vi "Prograss Bar Caller.vi"(8 "error in":errorcluster, 10 "Progress bar window values input":T1) -> (0 "error out":errorcluster)   [LabVIEW 2020]
uses:
  Progress bar window values input cluster.ctl
  Global Variables/General Globals.vi
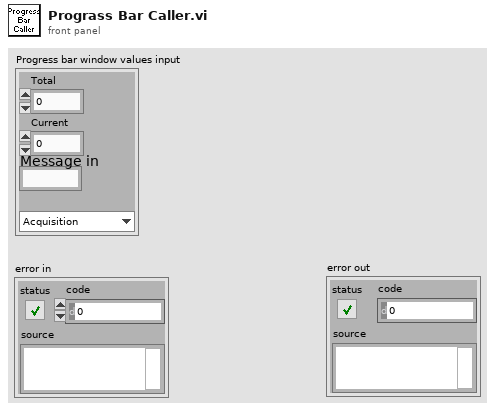
[diagram p1: front panel]
types:
  T1 = typedef "Progress bar window values input cluster.ctl" = cluster{"Total":i32, "Current":i32, "Message in":string, "Sender":enum16{"Acquisition", "Logging", "File gen"}}
  T2 = typedef "Progressbar window queue ref.ctl" = refnum<queue>
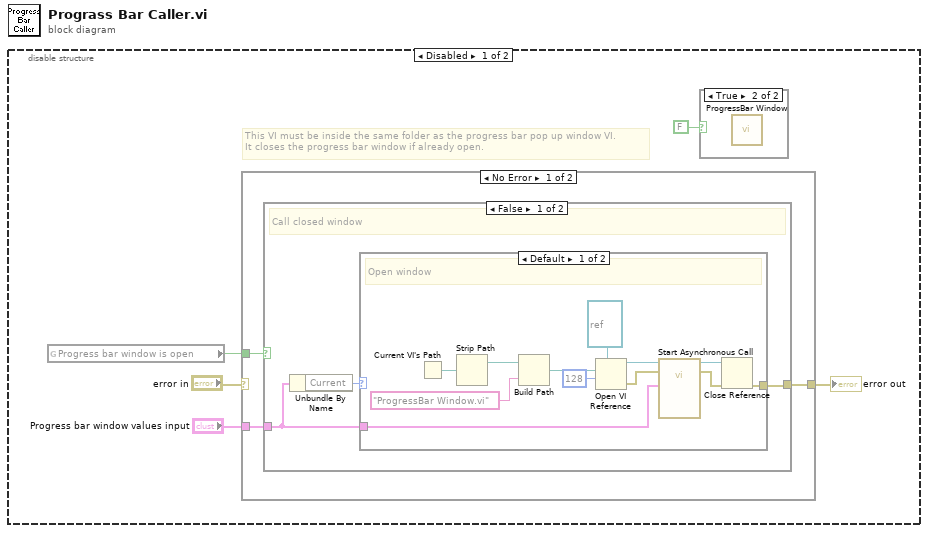
[diagram p0: block diagram]
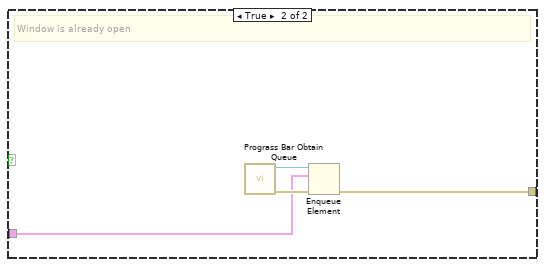
[diagram p3: hidden frame]
diagram:
  n1 = disable-structure shown="Disabled" {
    frame Disabled {
      # "This VI must be inside the same folder as the progress bar pop up window VI.\nIt closes the progress bar window if already open."
      n2 = global read "General Globals.vi" "Progress bar window is open"() -> (w1:bool)
      n3 = case shown="No Error" "error in" {
        selector: "error in" -> [_ w28]
        tunnel: "Progress bar window values input" -> [w8 _]
        tunnel: w1 -> [w7 _]
        tunnel: [w6 w28] -> w3
        frame No Error {
          n4 = case shown="False" w7 {
            tunnel: w8 -> [w10 w24]
            tunnel: [w11 w27] -> w6
            frame False {
              # "Call closed window"
              n5 = Unbundle By Name(w10) -> ("Current"=w9:i32)
              n6 = case shown="Default" w9 {
                tunnel: [w13 _] -> w11
                tunnel: w10 -> [w12 _]
                frame Default {
                  # "Open window"
                  n7 = Current VI's Path() -> (path=w21:path)
                  n8 = Strip Path(path=w21) -> (stripped path=w20:path)  [unwired: 1 out]
                  n9 = Build Path(base path=w20, name or relative path="ProgressBar Window.vi") -> (appended path=w18:path)
                  n10 = Open VI Reference(type specifier VI Refnum (for type only)=refnum<vi> refnum, vi path=w18, options=128) -> (vi reference=w17:refnum<vi>, error out=w14:errorcluster)  [unwired: 3 in]
                  n11 = call-by-ref "Start Asynchronous Call"(reference=w17, error in=w14, "Progress bar window values input cluster"=w12) -> (reference out=w16:refnum<vi>, error out=w15:errorcluster)  [unwired: 10 in, 1 out]
                  n12 = Close Reference(reference=w16, error in (no error)=w15) -> (error out=w13:errorcluster)
                }
                frame -2 {
                  # "Do not open. Already closed."
                }
              }
            }
            frame True {
              # "Window is already open"
              n13 = call "Prograss Bar Obtain Queue.vi"() -> ("error out"=w25:errorcluster, "Progressbar window queue ref"=w26:T2)  [unwired: 10 in]
              n14 = Enqueue Element(queue=w26, element=w24, error in (no error)=w25) -> (error out=w27:errorcluster)  [unwired: 1 in, 2 out]
            }
          }
        }
        frame Error {
        }
      }
      "error out" <- w3
      n15 = case shown="True" FALSE {
        frame False {
        }
        frame True {
          n16 = call "ProgressBar Window.vi"() -> ()  [unwired: 11 in, 1 out]
        }
      }
    }
    frame Enabled {
    }
  }
